vi "Generate New Message Libary Project.vi"() -> ()   [LabVIEW 2017]
panel:
  in  "Destination Directory":path
  in  "Hardware Device Name":string
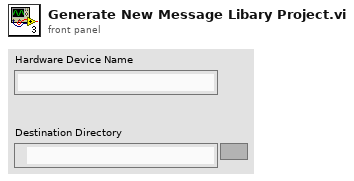
[diagram p1: front panel]
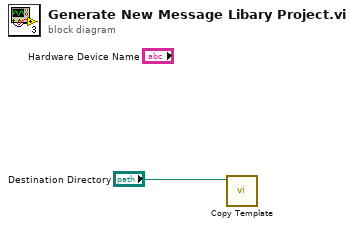
[diagram p0: block diagram]
diagram:
  n1 = call "Copy Template.vi"("Destination Directory"="Destination Directory") -> ()  [unwired: 9 in, 2 out]
